vi "DFD Filtering (Array NChan).vi"(7 "init? (F)":bool, 8 "error in (no error)":errorcluster, 10 "filter":T1={"mSRate_Fs"=1.0, "mSRate_Version"="2.0", "mSRate_Comments"="", "mSRate_OrgCoef"={"type"=enum."Undefined", "gain"=1.0, "coef a (k)"=[], "coef b (v)"=[]}, "mSRate_CurCoef"={"type"=enum."Undefined", "gain"=1.0, "coef a (k)"=[], "coef b (v)"=[]}, "mSRate_Quantized?"=FALSE, "mSRate_QCoef"={"type"=enum."Undefined", "gain"=1.0, "coef a (k)"=[], "coef b (v)"=[]}, "mSRate_QSettings"=[], "mSRate_Order"=0, "mSRate_Scaling"={"mSRate_ScaleByPowerOf2?"=FALSE, "mSRate_ScaleType"=enum."No Norm"}} {"mSRate_QSettings"."source" items=["Coef a/k"=0, "Coef b/v"=7, "Input"=1, "Output"=2, "Multiplicand"=3, "Product"=4, "Sum"=5, "Delay"=6, "Gain"=8]}, 11 "signal in":dbl[][](array[numeric])) -> (0 "error out":errorcluster, 3 "signal out":dbl[][](array[numeric]))   [LabVIEW 2017, in "NI_DigFilterLicensed.lvlib"]
doc: "Filters an input signal continuously. Wire data to the <B>signal in</B> input to determine the polymorphic instance to use or manually select the instance."
uses:
  <vilib>/addons/Digital Filter Design/NI_DigFilterLicensed.lvlib
  <vilib>/addons/Digital Filter Design/_Objects.llb/DFD Filter Obj.ctl
  <vilib>/addons/Digital Filter Design/_Objects.llb/DFD Filter Coef.ctl
  <vilib>/addons/Digital Filter Design/_Objects.llb/DFD Filter Structure Type Selector.ctl
  <vilib>/addons/Digital Filter Design/_Objects.llb/dfd_Internal Quantization Settings.ctl
  <vilib>/addons/Digital Filter Design/_Objects.llb/dfd_Internal Quantization Srcs.ctl
  <vilib>/addons/Digital Filter Design/_Objects.llb/DFD Coef Norm Type.ctl
  <vilib>/addons/Digital Filter Design/NI_DigFilter_Process.lvlib
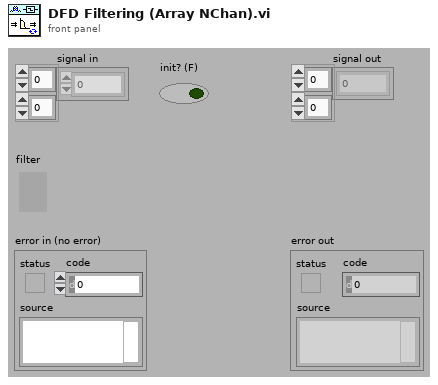
[diagram p1: front panel]
types:
  T1 = typedef "NI_DigFilterLicensed.lvlib/DFD Filter Obj.ctl" = cluster{"mSRate_Fs":dbl, "mSRate_Version":string, "mSRate_Comments":string, "mSRate_OrgCoef":T2, "mSRate_CurCoef":T2, "mSRate_Quantized?":bool, "mSRate_QCoef":T2, "mSRate_QSettings":T4[], "mSRate_Order":i32, "mSRate_Scaling":cluster{"mSRate_ScaleByPowerOf2?":bool, "mSRate_ScaleType":T6}}
  T2 = typedef "NI_DigFilterLicensed.lvlib/DFD Filter Coef.ctl" = cluster{"type":T3, "gain":dbl, "coef a (k)":dbl[], "coef b (v)":dbl[]}
  T3 = typedef "NI_DigFilterLicensed.lvlib/DFD Filter Structure Type Selector.ctl" = enum16{"Undefined", "FIR Direct Form", "FIR Direct Form Transposed", "FIR Symmetric", "FIR Antisymmetric", "IIR Direct Form I", "IIR Direct Form I Transposed", "IIR Direct Form II", "IIR Direct Form II Transposed", "IIR Cascaded Second Order Sections Form I", "IIR Cascaded Second Order Sections Form I Transposed", "IIR Cascaded Second Order Sections Form II", "IIR Cascaded Second Order Sections Form II Transposed", "Lattice Allpass (basic sections)", "Lattice Allpass (one multiplier sections)", "Lattice Allpass (normalized sections)", "Lattice AR (basic sections)", "Lattice AR (one multiplier sections)", "Lattice AR (normalized sections)", "Lattice MA (minimum phase)", "Lattice MA (maximum phase)", "Lattice ARMA (basic sections)", "Lattice ARMA (one multiplier sections)", "Lattice ARMA (normalized sections)"}
  T4 = typedef "NI_DigFilterLicensed.lvlib/dfd_Internal Quantization Settings.ctl" = cluster{"source":T5, "wl":i16, "iwl":i16, "overflow mode":enum16{"Saturation", "Wrap"}, "rounding mode":enum16{"Nearest", "Truncation"}, "signed?":bool}
  T5 = typedef "NI_DigFilterLicensed.lvlib/dfd_Internal Quantization Srcs.ctl" = u16
  T6 = typedef "NI_DigFilterLicensed.lvlib/DFD Coef Norm Type.ctl" = enum16{"No Norm", "Time Domain 1-Norm", "Time Domain 2-Norm", "Time Domain Inf-Norm"}
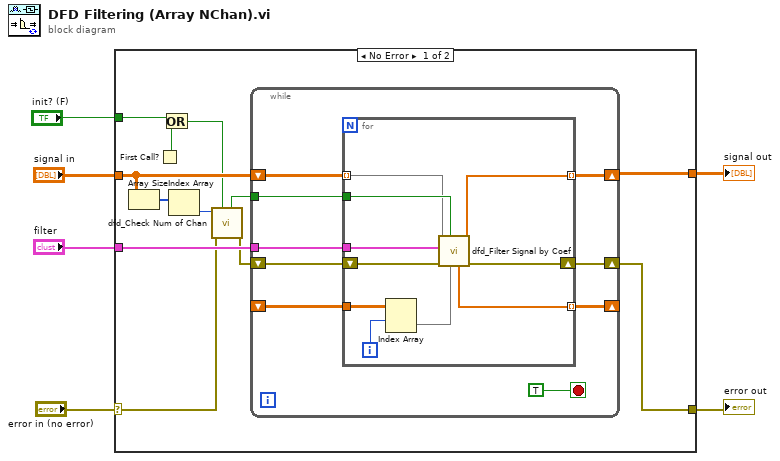
[diagram p0: block diagram]
diagram:
  n1 = case shown="No Error" "error in (no error)" {
    selector: "error in (no error)" -> [w8 w38]
    tunnel: [w17 w38] -> w4
    tunnel: "filter" -> [w18 _]
    tunnel: "signal in" -> [w13 _]
    tunnel: [w16 _] -> w2
    tunnel: "init? (F)" -> [w14 _]
    frame No Error {
      n2 = Array Size(array=w13) -> (size(s)=w12:i32[])
      n3 = First Call?() -> (First Call?: T/F=w15:bool)
      n4 = Or(x=w14, y=w15) -> (x .or. y?=w10:bool)
      n5 = Index Array(array=w12) -> (element=w11:i32)  [unwired: 1 in]
      n6 = call <vilib>:"dfd_Check Num of Chan.vi"("init in"=w10, "error in (no error)"=w8, "#ch in"=w11) -> ("error out"=w7:errorcluster, "init out"=w9:bool)  [unwired: 7 out]
      n7 = while {
        tunnel: w18 -> [w26]
        shift-right: [w20] -> _
        shift-left: _ -> [w19]
        tunnel: w9 -> [w23]
        shift-right: [w24] -> w16
        shift-left: w13 -> [w21]
        shift-right: [w22] -> w17
        shift-left: w7 -> [w25]
        stop <- TRUE stop-if-true
        n8 = for {
          tunnel: w26 -> [w37]
          shift-right: [w34] -> w22
          shift-left: w25 -> [w36]
          tunnel: w23 -> [w35]
          tunnel: w21 -> [w33] mode=indexing
          tunnel: [w32] -> w24 mode=indexing
          tunnel: w19 -> [w30]
          tunnel: [w31] -> w20 mode=indexing
          i -> [w29]
          n9 = Index Array(array=w30, index (row)=w29) -> (element=w28:dbl[])  [unwired: 1 in]
          n10 = call <vilib>:"dfd_Filter Signal by Coef.vi"("state in"=w28, "initH?"=w35, "error in(no error)"=w36, "filter"=w37, "x"=w33) -> ("error out"=w34:errorcluster, "filtered x"=w32:dbl[], "state out"=w31:dbl[])  [unwired: 1 in, 3 out]
        }
      }
    }
    frame Error {
    }
  }
  "error out" <- w4
  "signal out" <- w2
